vi "set current(SubVI).vi"(0 "源":i32, 1 "参考信号 1":T2, 2 "参考信号 3":T2, 5 "仪器设置":T1, 7 "电流":dbl, 9 "频率":dbl, 11 "电阻":dbl, 12 "参考信号2":T2, 13 "Voltage/curent Level":dbl, 14 "参考信号 4":T2) -> (10 "电压":dbl)   [LabVIEW 2019, in "old.lvlib"]
uses:
  old.lvlib
  lib/Keithley 622x/Configure/6221 Wave/Low Level/Typedefs/KE6221 -- Wave Type.ctl
  lib/Keithley 622x/Configure/Source/Typedefs/KE622x -- Current Level.ctl
  lib/Keithley 622x/Configure/6221 Wave/Low Level/Typedefs/KE6221 -- Wave Playback Time.ctl
  lib/Keithley 622x/Configure/6221 Wave/Low Level/Typedefs/KE6221 -- Wave Ranging Mode.ctl
  lib/Stanford Research 830/Stanford Research 830.lvlib
  lib/Keithley 622x/Keithley 622x.lvlib
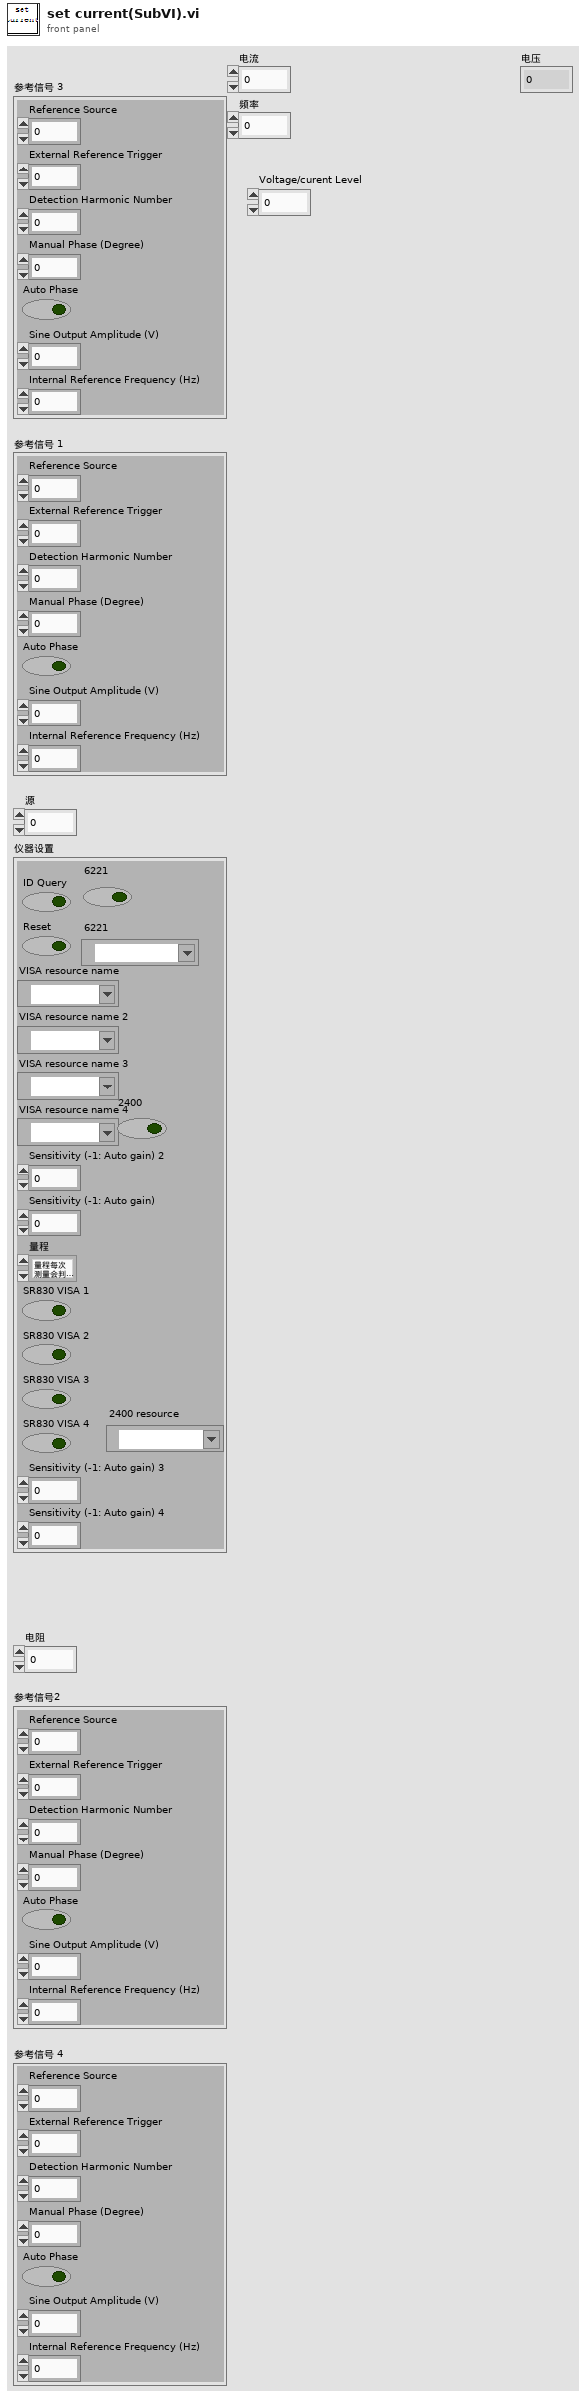
[diagram p1: front panel]
types:
  T1 = cluster{"ID Query":bool, "Reset":bool, "VISA resource name":refnum<visa-resource-name>, "VISA resource name 2":refnum<visa-resource-name>, "VISA resource name 3":refnum<visa-resource-name>, "VISA resource name 4":refnum<visa-resource-name>, "Sensitivity (-1: Auto gain) 2":i16, "Sensitivity (-1: Auto gain)":i16, "量程":enum16{"量程每次测量会判定", "量程不变为设定值"}, "SR830 VISA 1":bool, "SR830 VISA 2":bool, "SR830 VISA 3":bool, "SR830 VISA 4":bool, "Sensitivity (-1: Auto gain) 3":i16, "Sensitivity (-1: Auto gain) 4":i16, "6221":bool, "6221":refnum<visa-resource-name>, "2400":bool, "2400 resource":refnum<visa-resource-name>}
  T2 = cluster{"Reference Source":u16, "External Reference Trigger  ":u16, "Detection Harmonic Number ":dbl, "Manual Phase (Degree)":dbl, "Auto Phase ":bool, "Sine Output Amplitude (V)":dbl, "Internal Reference Frequency (Hz)":dbl}
  T3 = typedef "Keithley 622x.lvlib/KE6221 -- Wave Ranging Mode.ctl" = enum16{"Best", "Fixed"}
  T4 = typedef "Keithley 622x.lvlib/KE6221 -- Wave Playback Time.ctl" = dbl
  T5 = typedef "Keithley 622x.lvlib/KE622x -- Current Level.ctl" = dbl
  T6 = typedef "Keithley 622x.lvlib/KE6221 -- Wave Type.ctl" = enum16{"Sinusoid", "Square", "Ramp", "Arbitrary 0", "Arbitrary 1", "Arbitrary 2", "Arbitrary 3", "Arbitrary 4"}
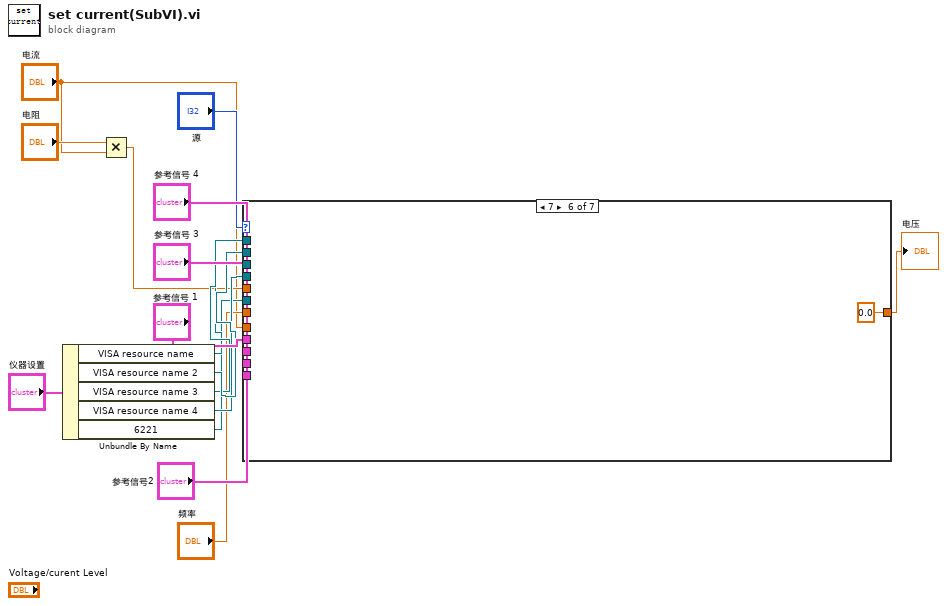
[diagram p0: block diagram]
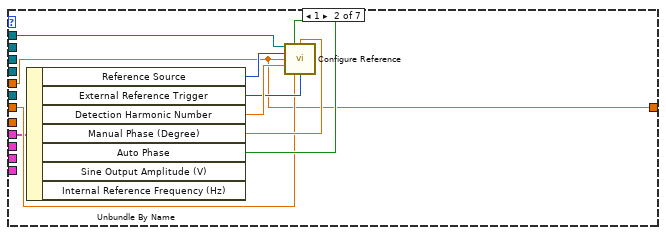
[diagram p3: hidden frame]
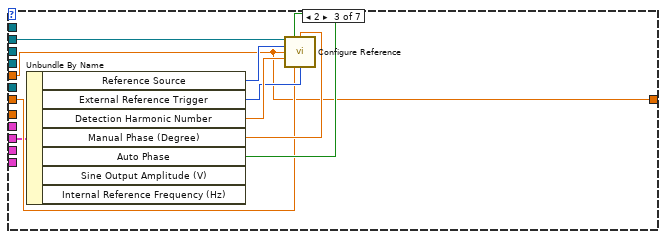
[diagram p4: hidden frame]
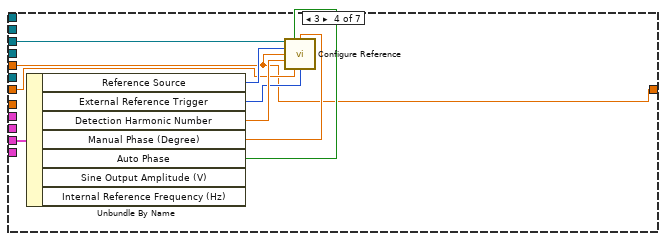
[diagram p5: hidden frame]
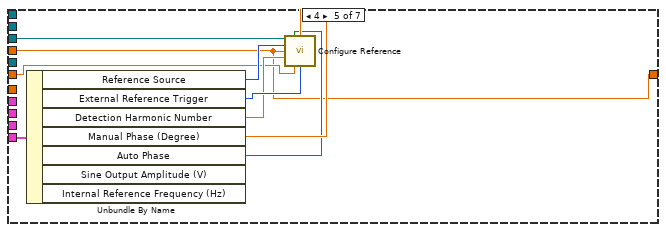
[diagram p6: hidden frame]
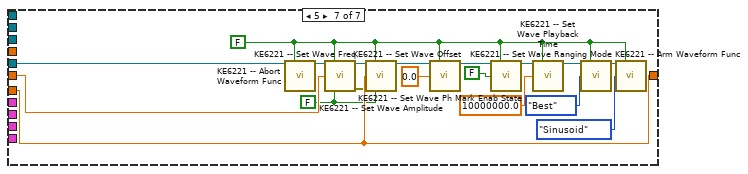
[diagram p7: hidden frame]
diagram:
  n1 = Unbundle By Name("仪器设置") -> ("VISA resource name"=w8:refnum<visa-resource-name>, "VISA resource name 2"=w11:refnum<visa-resource-name>, "VISA resource name 3"=w10:refnum<visa-resource-name>, "VISA resource name 4"=w9:refnum<visa-resource-name>, "6221"=w3:refnum<visa-resource-name>)
  n2 = Multiply(x="电阻", y="电流") -> (x*y=w7:dbl)
  n3 = case shown="7" "源" {
    tunnel: w7 -> [w17 w18 w27 w36 w45 _ _]
    tunnel: "频率" -> [_ w21 w29 w38 w47 _ w70]
    tunnel: w8 -> [_ w20 _ _ _ _ _]
    tunnel: w9 -> [_ _ _ _ w48 _ _]
    tunnel: w10 -> [_ _ _ w39 _ _ _]
    tunnel: w11 -> [_ _ w30 _ _ _ _]
    tunnel: "参考信号 1" -> [_ w19 _ _ _ _ _]
    tunnel: "参考信号2" -> [_ _ w28 _ _ _ _]
    tunnel: "参考信号 3" -> [_ _ _ w37 _ _ _]
    tunnel: "参考信号 4" -> [_ _ _ _ w46 _ _]
    tunnel: w3 -> [_ _ _ _ _ _ w67]
    tunnel: "电流" -> [_ _ _ _ _ _ w71]
    tunnel: [w17 w18 w27 w36 w45 0.0 ("电流") w71] -> w1
    frame 0, Default {
    }
    frame 1 {
      n4 = Unbundle By Name(w19) -> ("Reference Source"=w26:u16, "External Reference Trigger"=w24:u16, "Detection Harmonic Number"=w25:dbl, "Manual Phase (Degree)"=w22:dbl, "Auto Phase"=w23:bool)  [unwired: 2 out]
      n5 = call "Configure Reference.vi"("VISA resource name"=w20, "Auto Phase (T: Enabled)"=w23, "Manual Phase (0 Degree)"=w22, "Reference Source (1: Internal)"=w26, "Sine Output Amplitude (1 V)"=w18, "Detection Harmonic Number (1)"=w25, "Internal Reference Frequency (1000 Hz)"=w21, "External Reference Trigger (0: Sine Zero Crossing)"=w24) -> ()  [unwired: 6 in, 2 out]
    }
    frame 2 {
      n6 = Unbundle By Name(w28) -> ("Reference Source"=w35:u16, "External Reference Trigger"=w33:u16, "Detection Harmonic Number"=w34:dbl, "Manual Phase (Degree)"=w31:dbl, "Auto Phase"=w32:bool)  [unwired: 2 out]
      n7 = call "Configure Reference.vi"("VISA resource name"=w30, "Auto Phase (T: Enabled)"=w32, "Manual Phase (0 Degree)"=w31, "Reference Source (1: Internal)"=w35, "Sine Output Amplitude (1 V)"=w27, "Detection Harmonic Number (1)"=w34, "Internal Reference Frequency (1000 Hz)"=w29, "External Reference Trigger (0: Sine Zero Crossing)"=w33) -> ()  [unwired: 6 in, 2 out]
    }
    frame 3 {
      n8 = Unbundle By Name(w37) -> ("Reference Source"=w44:u16, "External Reference Trigger"=w42:u16, "Detection Harmonic Number"=w43:dbl, "Manual Phase (Degree)"=w40:dbl, "Auto Phase"=w41:bool)  [unwired: 2 out]
      n9 = call "Configure Reference.vi"("VISA resource name"=w39, "Auto Phase (T: Enabled)"=w41, "Manual Phase (0 Degree)"=w40, "Reference Source (1: Internal)"=w44, "Sine Output Amplitude (1 V)"=w36, "Detection Harmonic Number (1)"=w43, "Internal Reference Frequency (1000 Hz)"=w38, "External Reference Trigger (0: Sine Zero Crossing)"=w42) -> ()  [unwired: 6 in, 2 out]
    }
    frame 4 {
      n10 = Unbundle By Name(w46) -> ("Reference Source"=w49:u16, "External Reference Trigger"=w51:u16, "Detection Harmonic Number"=w50:dbl, "Manual Phase (Degree)"=w53:dbl, "Auto Phase"=w52:bool)  [unwired: 2 out]
      n11 = call "Configure Reference.vi"("VISA resource name"=w48, "Auto Phase (T: Enabled)"=w52, "Manual Phase (0 Degree)"=w53, "Reference Source (1: Internal)"=w49, "Sine Output Amplitude (1 V)"=w45, "Detection Harmonic Number (1)"=w50, "Internal Reference Frequency (1000 Hz)"=w47, "External Reference Trigger (0: Sine Zero Crossing)"=w51) -> ()  [unwired: 6 in, 2 out]
    }
    frame 7 {
    }
    frame 5 {
      w68 = FALSE ("Read Back Set Value? (T)")
      w55 = FALSE ("Check For SCPI Errors? (T)")
      n12 = call "KE6221 -- Abort Waveform Func.vi"("Resource In"=w67, "Check For SCPI Errors? (T)"=w55) -> ("Resource Out (dupl)"=w66:refnum<visa-resource-name>)  [unwired: 12 in, 1 out]
      n13 = call "KE6221 -- Set Wave Freq.vi"("Resource In"=w66, "Check For SCPI Errors? (T)"=w55, "Wave Frequency In (Hz)"=w70, "Read Back Set Value? (T)"=w68) -> ("Resource Out (dupl)"=w72:refnum<visa-resource-name>, "error out"=w69:errorcluster)  [unwired: 9 in, 1 out]
      n14 = call "KE6221 -- Set Wave Amplitude.vi"("Resource In"=w72, "Check For SCPI Errors? (T)"=w55, "Wave Amplitude In"=w71, "error in (no error)"=w69, "Read Back Set Value? (T)"=w68) -> ("Resource Out (dupl)"=w64:refnum<visa-resource-name>)  [unwired: 8 in, 2 out]
      n15 = call "KE6221 -- Set Wave Offset.vi"("Resource In"=w64, "Check For SCPI Errors? (T)"=w55, "Wave Offset In (A)"=T5 0.0) -> ("Resource Out (dupl)"=w62:refnum<visa-resource-name>)  [unwired: 10 in, 2 out]
      n16 = call "KE6221 -- Set Wave Ph Mark Enab State.vi"("Resource In"=w62, "Check For SCPI Errors? (T)"=w55, "Phase Marker Enabled?"=FALSE) -> ("Resource Out (dupl)"=w60:refnum<visa-resource-name>)  [unwired: 11 in, 1 out]
      n17 = call "KE6221 -- Set Wave Playback Time.vi"("Resource In"=w60, "Check For SCPI Errors? (T)"=w55, "Playback Time (s) In"=T4 10000000.0) -> ("Resource Out (dupl)"=w58:refnum<visa-resource-name>)  [unwired: 10 in, 2 out]
      n18 = call "KE6221 -- Set Wave Ranging Mode.vi"("Resource In"=w58, "Check For SCPI Errors? (T)"=w55, "Ranging Mode"=KE6221_--_Wave_Ranging_Mode."Best") -> ("Resource Out (dupl)"=w56:refnum<visa-resource-name>)  [unwired: 11 in, 1 out]
      n19 = call "KE6221 -- Arm Waveform Func.vi"("Resource In"=w56, "Check For SCPI Errors? (T)"=w55, "Wave Type"=KE6221_--_Wave_Type."Sinusoid") -> ()  [unwired: 11 in, 2 out]
    }
  }
  "电压" <- w1
